vi "Signal Start and Length.vi"(0 "Time Signal IN":dbl[](array[numeric])) -> (14 "Start Index":i32, 15 "Length":i32)   [LabVIEW 2020, in "TEXT.lvclass"]
uses:
  TEXT.lvclass
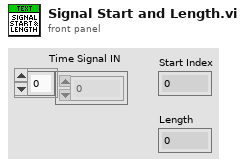
[diagram p1: front panel]
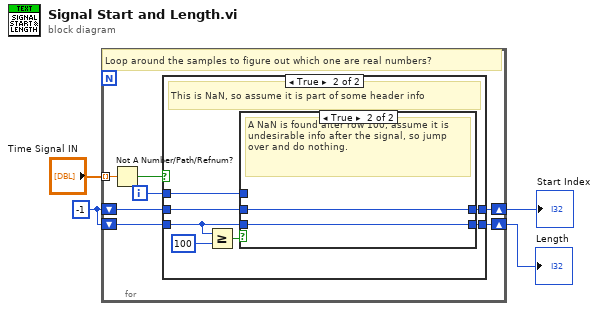
[diagram p0: block diagram]
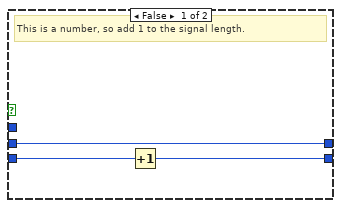
[diagram p2: hidden frame]
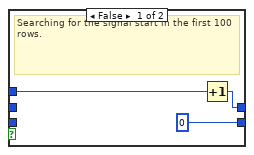
[diagram p3: hidden frame]
diagram:
  w1 = -1
  n1 = for {
    shift-right: [w11] -> w3
    shift-left: w1 -> [w8]
    shift-right: [w9] -> w2
    shift-left: w1 -> [w7]
    tunnel: "Time Signal IN" -> [w5] mode=indexing
    i -> [w10]
    # "Loop around the samples to figure out which one are real numbers?"
    n2 = Not A Number/Path/Refnum?(number/path/refnum=w5) -> (NaN/Path/Refnum?=w6:bool)
    n3 = case shown="True" w6 {
      tunnel: [w14 w20] -> w11
      tunnel: w10 -> [_ w21]
      tunnel: [w12 w19] -> w9
      tunnel: w8 -> [w14 w16]
      tunnel: w7 -> [w13 w15]
      frame False {
        # "This is a number, so add 1 to the signal length."
        n4 = Increment(x=w13) -> (x+1=w12:i32)
      }
      frame True {
        # "This is NaN, so assume it is part of some header info"
        n5 = Greater Or Equal?(x=w15, y=100) -> (x >= y?=w18:bool)
        n6 = case shown="True" w18 {
          tunnel: w21 -> [w24 _]
          tunnel: [w23 w26] -> w20
          tunnel: [0 w25] -> w19
          tunnel: w16 -> [_ w26]
          tunnel: w15 -> [_ w25]
          frame False {
            # "Searching for the signal start in the first 100 rows."
            n7 = Increment(x=w24) -> (x+1=w23:i32)
          }
          frame True {
            # "A NaN is found after row 100, assume it is undesirable info after the signal, so jump over and do nothing."
          }
        }
      }
    }
  }
  "Start Index" <- w3
  "Length" <- w2
